vi "edit.vi"(8 "error in (no error)":errorcluster, 11 "TCSettings in":refnum<class "TCSettings.lvclass">) -> (0 "error out":errorcluster, 2 "cancelIsTrue out":bool, 3 "TCSettings out":refnum<class "TCSettings.lvclass">)   [LabVIEW 2016, in "Settings.lvlib" / "TCSettings.lvclass"]
uses:
  TCSettings.lvclass
  ConfigurationTC/ConfigurationTypedefs/Set/ExampleSettings.ctl
  home/harini/tcs/ts_sedspectrometer/Settings/Settings/Setting.lvclass
  ConfigurationTC/ConfigurationTypedefs/Base/CommunicationConfig.ctl
  ConfigurationTC/ConfigurationTypedefs/Base/LoopConfig.ctl
  ConfigurationTC/ConfigurationTypedefs/Base/BaseSALSettings.ctl
  Settings/Setting.lvclass/Setting.ctl
  <vilib>/Utility/xml.llb/Write to XML File(string).vi
  Settings/Setting.lvclass
  ConfigurationTC/ConfigurationTypedefs/ConfigurationTypedefs.lvlib
panel:
  in  "SettingTab":T1(tab)
  in  "HPSettings":T2
  in  "SALSettings":T3={"IPAddress"="127.0.0.1", "Port"=0, "StartupScript"="source /usr/ts_sal/setup.env && /usr/ts_sal/test/m1m3/cpp/src/SALPipe %d -1"}
  in  "loopConfig":T4={"hostLoopPeriod_s"=0.016, "hostLoopPeriodAllowedJitter_percent"=10.0} {"hostLoopPeriodAllowedJitter_percent" min=1.0 max=100.0; "hostLoopPeriod_s" min=0.001 max=600.0}
  in  "communicationConfig":T5 {"InstanceIdentifier" min=-1}
  out "String":string
  in  "cancelIsTrue":bool
  in  "saveIsTrue":bool
  in  "Listbox":i32(listbox)
  # "(-1 for none)"
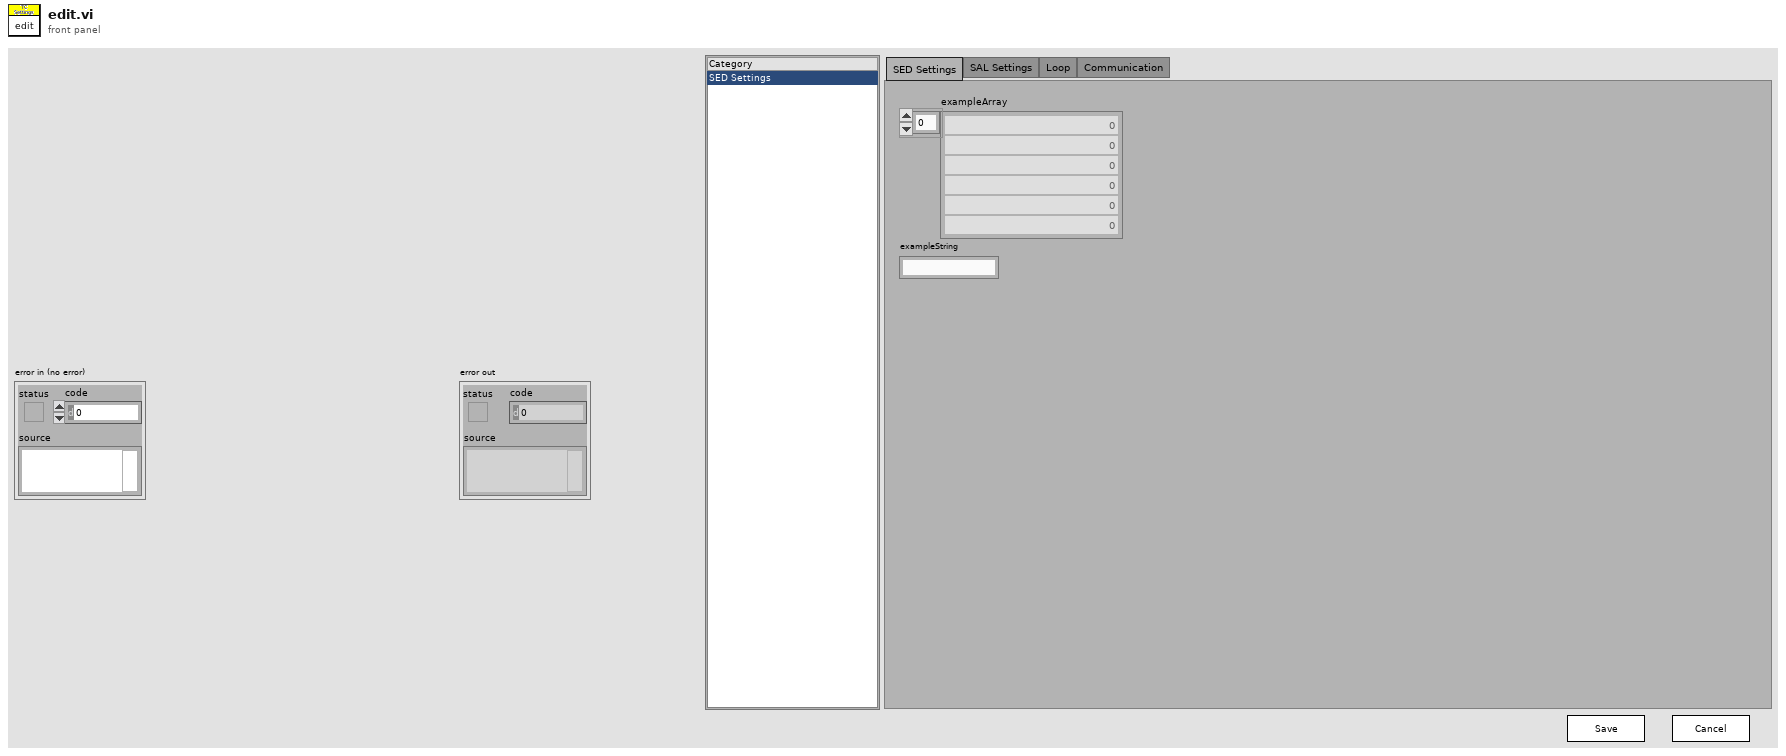
[diagram p1: front panel]
types:
  T1 = enum32{"SED Settings", "SAL Settings", "Loop", "Communication"}
  T2 = typedef "ConfigurationTypedefs.lvlib/ExampleSettings.ctl" = cluster{"exampleArray":i32[], "exampleString":string}
  T3 = typedef "ConfigurationTypedefs.lvlib/BaseSALSettings.ctl" = cluster{"IPAddress":string, "Port":u16, "StartupScript":string}
  T4 = typedef "ConfigurationTypedefs.lvlib/LoopConfig.ctl" = cluster{"hostLoopPeriod_s":dbl, "hostLoopPeriodAllowedJitter_percent":dbl}
  T5 = typedef "ConfigurationTypedefs.lvlib/CommunicationConfig.ctl" = cluster{"hostComputerAddress":string, "ComponentAcronym":string, "InstanceIdentifier":i32}
  T6 = enum32{"Invalid", "Standard", "Closed", "Hidden", "Minimized", "Maximized"}
  T7 = enum16{"open", "replace", "create", "open or create", "replace or create", "replace or create with confirmation"}
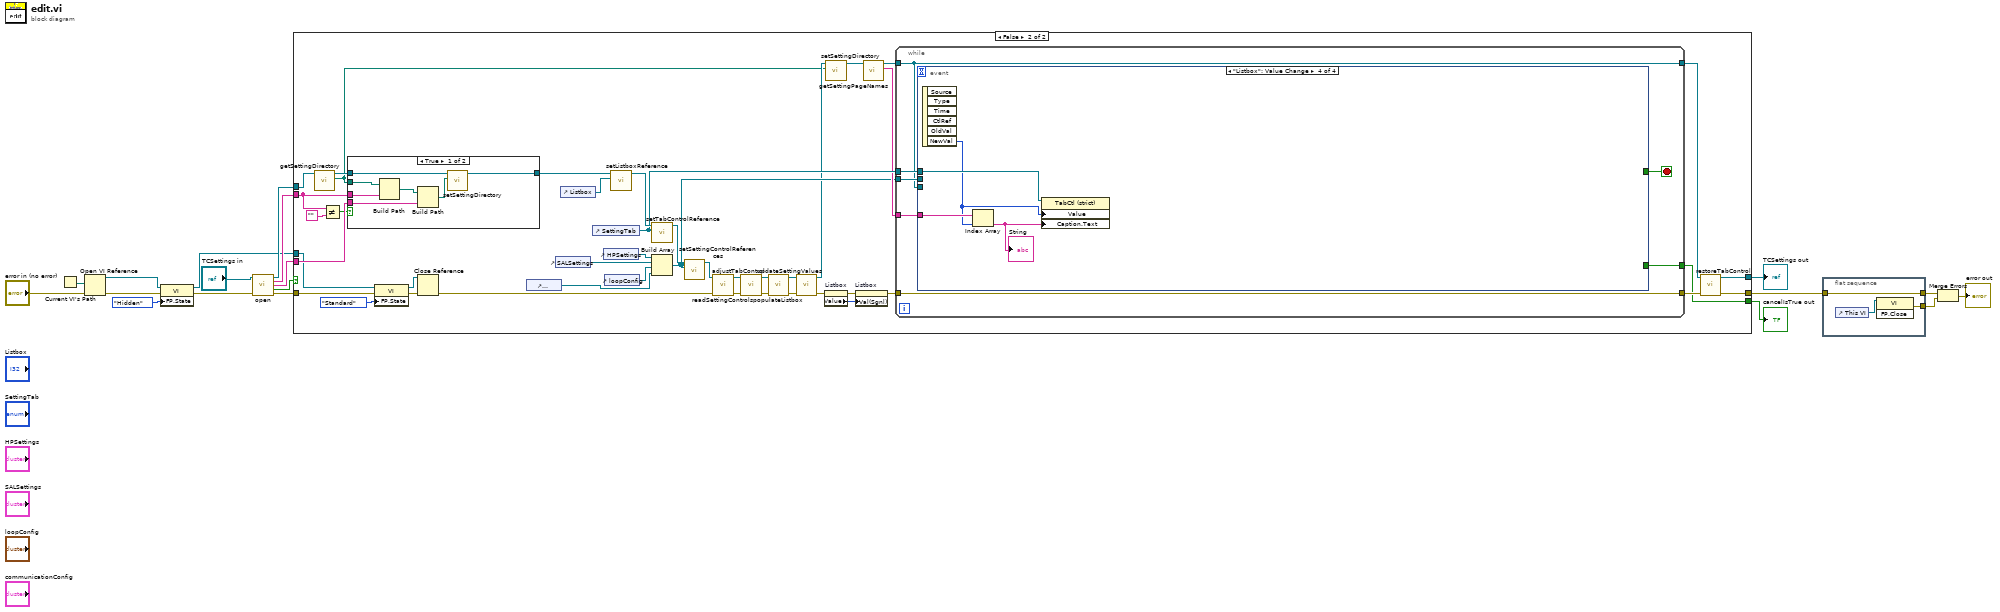
[diagram p0: block diagram]
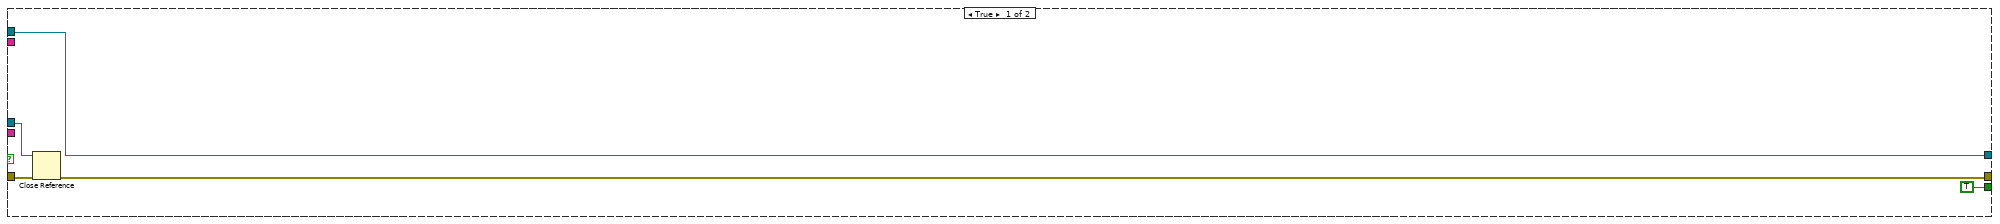
[diagram p2: hidden frame]
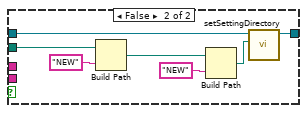
[diagram p3: hidden frame]
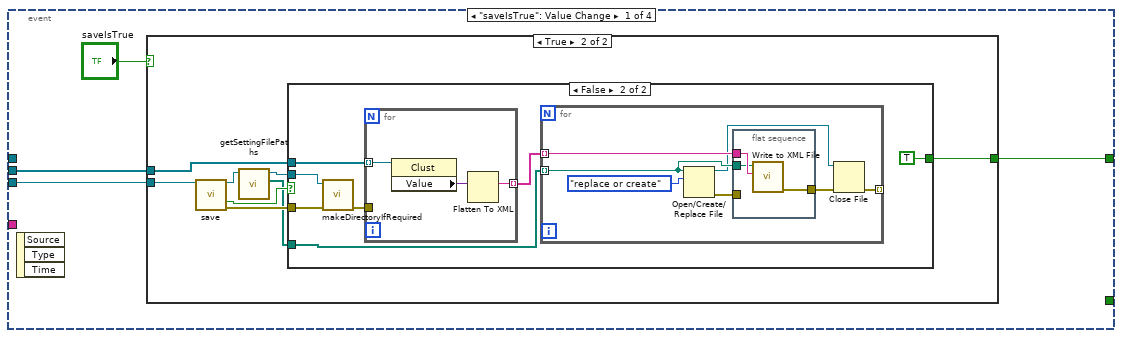
[diagram p4: hidden frame]
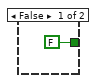
[diagram p5: hidden frame]
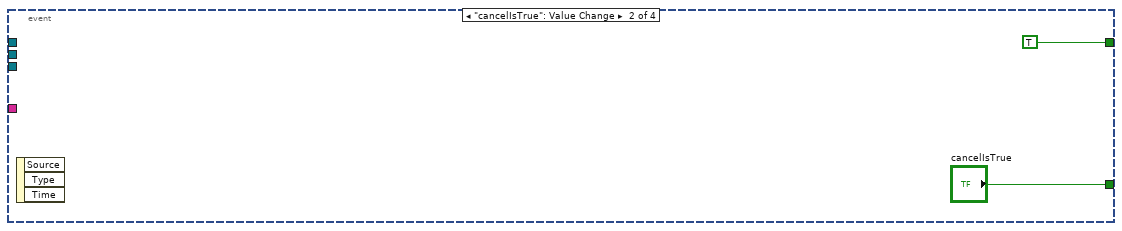
[diagram p7: hidden frame]
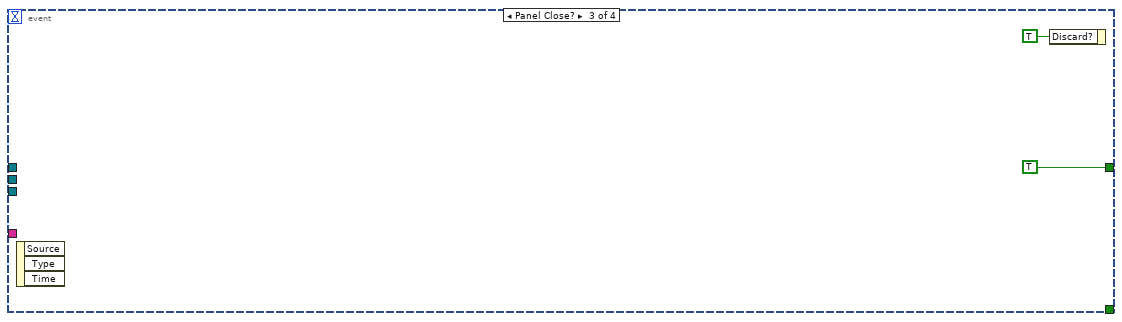
[diagram p8: hidden frame]
diagram:
  n1 = Current VI's Path() -> (path=w8:path)
  n2 = Open VI Reference(vi path=w8, error in (no error)="error in (no error)") -> (vi reference=w7:refnum<vi>, error out=w6:errorcluster)  [unwired: 4 in]
  n3 = property class="VI"(reference=w7, error in=w6, "FP.State"=T6."Hidden" ("Front Panel Window:State")) -> (reference out=w1:refnum<vi>, error out=w3:errorcluster)
  n4 = call "open.vi"("TCSettings in"="TCSettings in", "error in (no error)"=w3) -> ("TCSettings out"=w19:refnum<class "TCSettings.lvclass">, "SelectedSet"=w13:string, "SelectedVersion"=w15:string, "Canceled"=w11:bool, "error out"=w2:errorcluster)  [unwired: 9 in]
  n5 = case shown="False" w11 {
    tunnel: w19 -> [w24 w59]
    tunnel: w15 -> [_ w43]
    tunnel: [w24 w42] -> w9
    tunnel: [w20 w41] -> w14
    tunnel: w13 -> [_ w39]
    tunnel: [TRUE ("cancelIsTrue") w34] -> w12
    tunnel: w2 -> [w21 w28]
    tunnel: w1 -> [w22 w27]
    frame True {
      n6 = Close Reference(reference=w22, error in (no error)=w21) -> (error out=w20:errorcluster)
    }
    frame False {
      n7 = call "getSettingDirectory.vi"("BaseSetting in"=w59) -> ("SettingDirectory"=w35:path, "BaseSetting out"=w58:refnum<class "TCSettings.lvclass">)  [unwired: 9 in]
      n8 = Not Equal?(x=w39, y="") -> (x != y?=w38:bool)
      n9 = case shown="True" w38 {
        tunnel: w58 -> [w74 w81]
        tunnel: [w73 w80] -> w44
        tunnel: w43 -> [w71 _]
        tunnel: w35 -> [w69 w77]
        tunnel: w39 -> [w68 _]
        frame True {
          n10 = Build Path(base path=w69, name or relative path=w68) -> (appended path=w72:path)
          n11 = Build Path(base path=w72, name or relative path=w71) -> (appended path=w70:path)
          n12 = call "setSettingDirectory.vi"("SettingDirectory"=w70, "BaseSetting in"=w74) -> ("BaseSetting out"=w73:refnum<class "TCSettings.lvclass">)  [unwired: 9 in]
        }
        frame False {
          n13 = Build Path(base path=w77, name or relative path="NEW") -> (appended path=w79:path)
          n14 = Build Path(base path=w79, name or relative path="NEW") -> (appended path=w78:path)
          n15 = call "setSettingDirectory.vi"("SettingDirectory"=w78, "BaseSetting in"=w81) -> ("BaseSetting out"=w80:refnum<class "TCSettings.lvclass">)  [unwired: 9 in]
        }
      }
      n16 = property class="VI"(reference=w27, error in=w28, "FP.State"=T6."Standard" ("Front Panel Window:State")) -> (reference out=w31:refnum<vi>, error out=w32:errorcluster)
      n17 = Close Reference(reference=w31, error in (no error)=w32) -> (error out=w29:errorcluster)
      n18 = control-ref of="communicationConfig"() -> (w25:refnum<vi>)
      n19 = control-ref of="SALSettings"() -> (w33:refnum<vi>)
      n20 = control-ref of="Listbox"() -> (w61:refnum<vi>)
      n21 = control-ref of="SettingTab"() -> (w51:refnum<vi>)
      n22 = control-ref of="HPSettings"() -> (w60:refnum<vi>)
      n23 = control-ref of="loopConfig"() -> (w26:refnum<vi>)
      n24 = call "setListboxReference.vi"("ListboxReference"=w61, "Setting in"=w44) -> ("Setting out"=w62:refnum<class "TCSettings.lvclass">)  [unwired: 9 in]
      n25 = call "setTabControlReference.vi"("TabControlReference"=w51, "Setting in"=w62) -> ("Setting out"=w63:refnum<class "TCSettings.lvclass">)  [unwired: 9 in]
      n26 = Build Array(w60, w33, w26, w25) -> (w48:refnum<vi>[])
      n27 = call "setSettingControlReferences.vi"("SettingControlReferences"=w48, "Setting in"=w63) -> ("Setting out"=w64:refnum<class "TCSettings.lvclass">)  [unwired: 9 in]
      n28 = call "readSettingControls.vi"("error in (no error)"=w29, "BaseSetting in"=w64) -> ("error out"=w54:errorcluster, "BaseSetting out"=w65:refnum<class "TCSettings.lvclass">)  [unwired: 8 in]
      n29 = call "adjustTabControl.vi"("error in (no error)"=w54, "BaseSetting in"=w65) -> ("error out"=w53:errorcluster, "BaseSetting out"=w66:refnum<class "TCSettings.lvclass">)  [unwired: 8 in]
      n30 = call "populateListbox.vi"("error in (no error)"=w53, "BaseSetting in"=w66) -> ("error out"=w52:errorcluster, "BaseSetting out"=w67:refnum<class "TCSettings.lvclass">)  [unwired: 8 in]
      n31 = call "updateSettingValues.vi"("error in (no error)"=w52, "BaseSetting in"=w67) -> ("error out"=w55:errorcluster, "BaseSetting out"=w37:refnum<class "TCSettings.lvclass">)  [unwired: 8 in]
      n32 = property on="Listbox" class="LstBox (strict)"(error in=w55) -> (error out=w57:errorcluster, "Value"=w56:i32)  [unwired: 1 in, 1 out]
      n33 = call "setSettingDirectory.vi"("SettingDirectory"=w35, "BaseSetting in"=w37) -> ("BaseSetting out"=w36:refnum<class "TCSettings.lvclass">)  [unwired: 9 in]
      n34 = property on="Listbox" class="LstBox (strict)"(error in=w57, "Val(Sgnl)"=w56) -> (error out=w47:errorcluster)  [unwired: 1 in, 1 out]
      n35 = call "getSettingPageNames.vi"("Setting in"=w36) -> ("SettingPageNames"=w49:string[], "Setting out"=w50:refnum<class "TCSettings.lvclass">)  [unwired: 9 in]
      n36 = while {
        tunnel: w51 -> [w86]
        tunnel: w48 -> [w88]
        tunnel: [w83] -> w45
        tunnel: w50 -> [w83]
        tunnel: w47 -> [w85]
        tunnel: [w85] -> w46
        tunnel: [w84] -> w34
        tunnel: w49 -> [w82]
        stop <- w87 stop-if-true
        n37 = event shown="[3] \"Listbox\": Value Change" {
          selector: _ -> [_ _ _ _]
          dyn-events: _ -> [_ _ _ _]
          timeout: _ -> [_ _ _ _]
          tunnel: [w90 TRUE TRUE _] -> w87
          tunnel: w82 -> [_ _ _ w128]
          tunnel: w86 -> [_ _ _ w129]
          tunnel: w88 -> [w92 _ _ _]
          tunnel: [_ "cancelIsTrue" _ _] -> w84
          tunnel: w83 -> [w91 _ _ _]
          event "saveIsTrue": Value Change {
            n38 = event-data() -> ()  [unwired: 1 in, 3 out]
            n39 = case shown="True" "saveIsTrue" {
              tunnel: w92 -> [_ w101]
              tunnel: w91 -> [_ w100]
              tunnel: [FALSE w98] -> w90
              frame False {
              }
              frame True {
                n40 = call "save.vi"("M1M3Settings in"=w100) -> ("M1M3Settings out"=w96:refnum<class "TCSettings.lvclass">, "Canceled"=w97:bool, "error out"=w99:errorcluster)  [unwired: 12 in]
                n41 = call "getSettingFilePaths.vi"("Setting in"=w96) -> ("SettingFilePaths"=w94:path[], "Setting out"=w95:refnum<class "TCSettings.lvclass">)  [unwired: 9 in]
                n42 = case shown="False" w97 {
                  tunnel: w94 -> [_ w108]
                  tunnel: w101 -> [_ w107]
                  tunnel: w95 -> [_ w104]
                  tunnel: w99 -> [_ w103]
                  tunnel: [_ TRUE] -> w98
                  frame True {
                  }
                  frame False {
                    n43 = call "makeDirectoryIfRequired.vi"("error in (no error)"=w103, "BaseSetting in"=w104) -> ("error out"=w105:errorcluster)  [unwired: 8 in, 1 out]
                    n44 = for {
                      tunnel: w107 -> [w121] mode=indexing
                      tunnel: [w119] -> w106 mode=indexing
                      tunnel: w105 -> [_]
                      n45 = property class="Clust"(reference=w121) -> ("Value"=w120:variant)  [unwired: 1 in, 2 out]
                      n46 = Flatten To XML(anything=w120) -> (xml string=w119:string)
                    }
                    n47 = for {
                      tunnel: w108 -> [w112] mode=indexing
                      tunnel: w106 -> [w115] mode=indexing
                      tunnel: [w109] -> _ mode=indexing
                      n48 = Open/Create/Replace File(file path (use dialog)=w112, operation (0:open)=T7."replace or create") -> (refnum out=w111:refnum<file>, error out=w113:errorcluster)  [unwired: 4 in, 1 out]
                      n49 = flat-sequence {
                        tunnel: w115 -> [w118]
                        tunnel: [w117] -> w110
                        tunnel: w113 -> [_]
                        tunnel: w112 -> [w116]
                        frame #0 {
                          n50 = call-poly <vilib>:"Write to XML File.vi"("XML Input"=w118, "XML File Path"=w116) -> ("error out"=w117:errorcluster)  [unwired: 7 in, 2 out]
                        }
                      }
                      n51 = Close File(refnum=w111, error in=w110) -> (error out=w109:errorcluster)  [unwired: 1 out]
                    }
                  }
                }
              }
            }
          }
          event "cancelIsTrue": Value Change {
            n52 = event-data() -> ()  [unwired: 1 in, 3 out]
          }
          event Panel Close? {
            n53 = event-data() -> ()  [unwired: 1 in, 3 out]
            n54 = event-data("Discard?"=TRUE) -> ()  [unwired: 1 in, 1 out]
          }
          event "Listbox": Value Change {
            n55 = event-data() -> ("NewVal"=w127:i32)  [unwired: 1 in, 5 out]
            n56 = Index Array(array=w128, index=w127) -> (element=w126:string)
            "String" <- w126
            n57 = property class="TabCtl (strict)"(reference=w129, "Value"=w127, "Caption.Text"=w126) -> ()  [unwired: 1 in, 2 out]
          }
        }
      }
      n58 = call "restoreTabControl.vi"("error in (no error)"=w46, "BaseSetting in"=w45) -> ("error out"=w41:errorcluster, "BaseSetting out"=w42:refnum<class "TCSettings.lvclass">)  [unwired: 8 in]
    }
  }
  "cancelIsTrue out" <- w12
  "TCSettings out" <- w9
  n59 = flat-sequence {
    tunnel: [w131] -> w18
    tunnel: [w130] -> w17
    tunnel: w14 -> [w130]
    frame #0 {
      n60 = control-ref of="This VI"() -> (w132:refnum<vi>)
      n61 = invoke class="VI" method="FP.Close"(reference=w132) -> (error out=w131:errorcluster)  [unwired: 2 in, 2 out]
    }
  }
  n62 = Merge Errors(w17, w18) -> (→"error out":errorcluster)
